vi "Grobal Variable_Next Frame.vi"() -> ()   [LabVIEW 2015]
panel:
  out "Next frame?_Global":bool
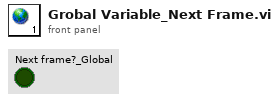
[diagram p1: front panel]
diagram:
